vi "monitor picoammeter.vi"() -> ()   [LabVIEW 2024]
uses:
  <vilib>/Platform/TimedLoop/XDataNode/timing_clust.ctl
  <vilib>/Platform/TimedLoop/XDataNode/nitl_modes.ctl
  <vilib>/Platform/TimedLoop/XDataNode/wakeup.ctl
  <vilib>/platform/TimedLoop/XDataNode/XDataNode.xnode
  <instrlib>/Keithley 648X Series/Keithley 648X Series.lvlib
  <vilib>/Platform/TimedLoop/XDataNode/XDNodeRunTimeDep.lvlib
panel:
  in  "Digital Filter Count (10)":i32=10
  out "Waveform Chart":dbl(graph)
  in  "stop":bool
  out "Measurement (nA)":dbl
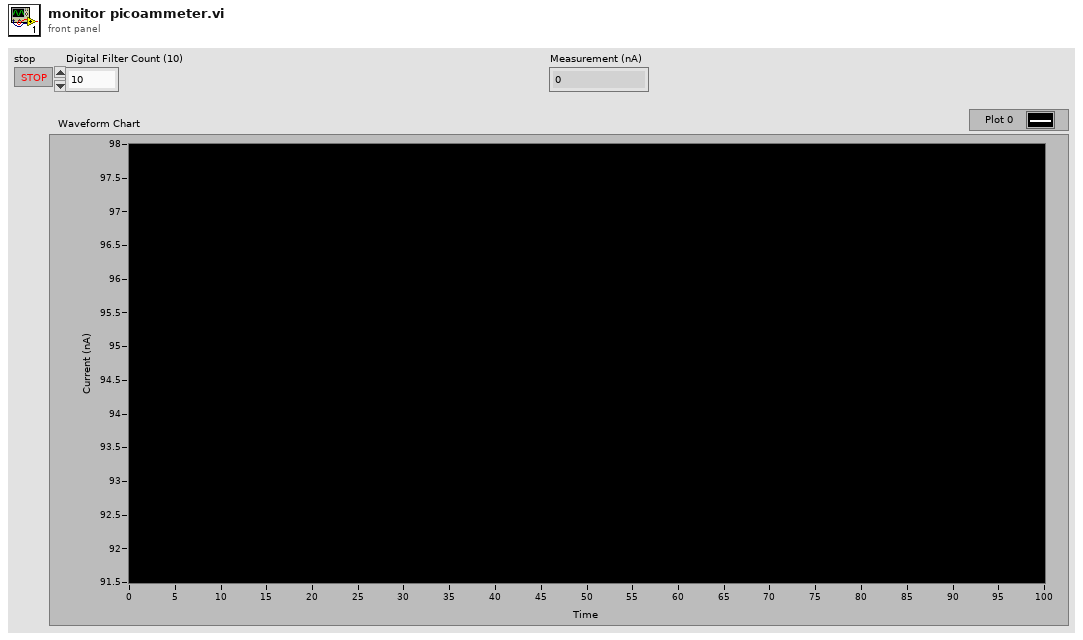
[diagram p1: front panel]
types:
  T1 = typedef "XDNodeRunTimeDep.lvlib/timing_clust.ctl" = cluster{"Expected End [f-1]":u64, "Actual End [f-1]":u64, "Finished Late? [f-1]":bool, "Expected End [i-1]":u64, "Actual End [i-1]":u64, "Finished Late? [i-1]":bool, "Expected Start [i]":u64, "Actual Start [i]":u64, "Expected Start [f]":u64, "Actual Start [f]":u64, "Source Name":string, "Structure Name":string, "Period":i64, "Deadline":i64, "Offset":i64, "Start":i64, "Priority":i32, "Timeout":i32, "Mode":T2, "Wakeup Reason":T3, "Error":errorcluster, "Source Type":string, "Secondary Source Type":string, "Global End Time":u64, "Global Start Time":u64, "Frame Duration":u64, "Iteration Duration":u64, "Assigned CPU":i32, "I/O Scan Engine Mode":u32}
  T2 = typedef "XDNodeRunTimeDep.lvlib/nitl_modes.ctl" = enum32{"No Change", "Process missed periods, maintain original phase", "Discard missed periods, maintain original phase", "Process missed periods, ignore original phase", "Discard missed periods, ignore original phase"}
  T3 = typedef "XDNodeRunTimeDep.lvlib/wakeup.ctl" = enum32{"Normal", "Aborted", "Asynchronous wakeup", "Timing source error", "Timed loop error", "Timeout"}
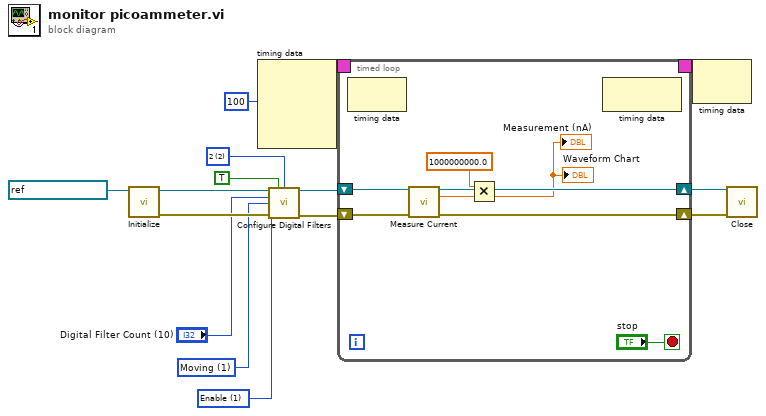
[diagram p0: block diagram]
diagram:
  w1 = u16 2 items=["1"=1, "2"=2, "3"=3, "4"=4, "5"=5] ("Median Filter Rank (1)")
  w4 = u16 1 items=["Repeating", "Moving"] ("Digital Filter Type (0: Repeating)")
  w5 = u16 1 items=["Disable", "Enable", "Advanced"] ("Enable Digital Filter (0: Disable)")
  n1 = call <instrlib>:"Initialize.vi"("VISA resource name"=refnum<visa-resource-name> "Picoammeter") -> ("error out"=w7:errorcluster, "VISA resource name out"=w9:refnum<visa-resource-name>)  [unwired: 9 in]
  n2 = node-c288(i64 100 ("Period")) -> (w12:T1)  [unwired: 3 in]
  n3 = call <instrlib>:"Configure Digital Filters.vi"("VISA resource name"=w9, "Enable Median Filter (F: Disable)"=TRUE, "Median Filter Rank (1)"=w1, "Digital Filter Count (10)"="Digital Filter Count (10)", "Digital Filter Type (0: Repeating)"=w4, "Enable Digital Filter (0: Disable)"=w5, "error in (no error)"=w7) -> ("VISA resource name out"=w8:refnum<visa-resource-name>, "error out"=w6:errorcluster)  [unwired: 7 in]
  n4 = timed-loop {
    timing: w12 -> [_]
    timing-out: [_] -> w11
    shift-right: [w22] -> w15
    shift-left: w6 -> [w23]
    shift-right: [w20] -> w14
    shift-left: w8 -> [w21]
    stop <- "stop" stop-if-true
    n5 = node-c288() -> ()  [unwired: 1 in, 1 out]
    n6 = call <instrlib>:"Measure Current.vi"("VISA resource name"=w21, "error in (no error)"=w23) -> ("VISA resource name out"=w20:refnum<visa-resource-name>, "Measurement"=w18:dbl, "error out"=w22:errorcluster)  [unwired: 11 in]
    n7 = Multiply(x=1000000000.0, y=w18) -> (x*y=→"Measurement (nA)" →"Waveform Chart":dbl)
    n8 = node-c288() -> ()  [unwired: 1 in, 1 out]
  }
  n9 = node-c288(w11) -> ()  [unwired: 1 out]
  n10 = call <instrlib>:"Close.vi"("error in (no error)"=w15, "VISA resource name"=w14) -> ()  [unwired: 9 in, 1 out]
